vi "Convert Error Cluster to Table.vi"(11 "Error Codes":cluster{i32, string}[](array[cluster])) -> (2 "Code":i32[](array[numeric]), 3 "String":string[](array[string]))   [LabVIEW 2019, in "OPC UA Client System Explorer.lvlib"] (continued)
running the VI, this error occurs. The most likely cause is that you added a new session, and tried to use that new session in a running VI. Solution: Configure all session in LabVIEW project, then run the VI(s) that use those sessions."}, {-1074384541, "NI-XNET:  (Hex 0xBFF63163) You used an empty name for an XNET database object (database, cluster, ECU, frame, or signal). Empty name is not supported. Solution: Refer to NI-XNET help for IO names to review the required syntax for the name, and change your code to use that syntax."}, {-1074384540, "NI-XNET:  (Hex 0xBFF63164) You used a name for an XNET database object (such as frame or signal) that did not include a valid cluster selection. Solution: Refer to the NI-XNET help for the IO name that you are using, and use the syntax specified for that class, which includes the cluster selection."}, {-1074384539, "NI-XNET:  (Hex 0xBFF63165) Unsupported database file version. Solution: Use only database versions that are supported by this version of NI-XNET. Please see the NI-XNET documentation for information on which database versions are currently supported."}, {-1074384538, "NI-XNET:  (Hex 0xBFF63166) You used an empty name for the XNET Session. Empty name is not supported. Solution: Use a valid XNET session name from your LabVIEW project."}, {-1074384537, "NI-XNET:  (Hex 0xBFF63167) There is not enough message RAM on the FlexRay hardware to configure the data partition for the object(s). Solution: Please refer to the manual for limitations on the number of objects that can be created at any given time based on the payload length."}, {-1074384536, "NI-XNET:  (Hex 0xBFF63168) The FlexRay keyslot ID has been configured and a startup session has been created. Either the keyslot ID needs to be configured OR the startup session needs to be created. Both cannot exist at the same time. Solution: Choose a single method to configure startup sessions in your application."}, {-1074384535, "NI-XNET:  (Hex 0xBFF63169) An unsupported session was created. For example, stream output is not supported on FlexRay hardware. Solution: Only use supported sessions in your application."}, {-1074384528, "NI-XNET:  (Hex 0xBFF63170) An XNET session was created after starting the Interface. Only the Stream Input session in the subordinate mode can be created after the Interface has started. Solution: Create sessions prior to starting the XNET Interface in your application."}, {-1074384527, "NI-XNET:  (Hex 0xBFF63171) The Single Slot property was enabled on the XNET FlexRay Interface after the interface had started. Solution: Enable the Single Slot property prior to starting the XNET FlexRay Interface."}, {-1074384526, "NI-XNET:  (Hex 0xBFF63172) The FlexRay macrotick offset specified for XNET Create Timing Source is unsupported. Example: Specifying a macrotick offset greater than MacroPerCycle will result in this error. Solution: Specify a macrotick offset within the supported range for the cluster."}, {-1074384525, "NI-XNET:  (Hex 0xBFF63173) You used invalid syntax in the name of a database object (signal, frame, or ECU). For example, you may have specified a frame's name as <cluster>.<frame>, which is allowed in NI-XNET for C/C++, but not NI-XNET for LabVIEW. Solution: Use the string syntax specified in the help topic for the XNET I/O name class you are using."}, {-1074384524, "NI-XNET:  (Hex 0xBFF63174) A LIN schedule entry name is ambiguous, e.g., a schedule entry with the same name exists in another schedule. Solution: Specify the schedule name for the schedule entry using the required syntax."}, {-1074384523, "NI-XNET:  (Hex 0xBFF63175) A LIN schedule entry with the same name already exists in the schedule. Solution: Use another name for this schedule entry."}, {-1074384522, "NI-XNET:  (Hex 0xBFF63176) At least one of the frames in the session has an undefined identifier. Solution: Set the frame's \"Identifier (Slot)\" property before creating the session."}, {-1074384521, "NI-XNET:  (Hex 0xBFF63177) At least one of the frames in the session has an undefined payload length. Solution: Set the frame's \"Payload Length (in bytes)\" property before creating the session."}, {-1074384520, "NI-XNET:  (Hex 0xBFF63178) At least one of the signals in the session has an undefined start bit. Solution: Set the \"Start Bit\" property of the signal before creating the session."}, {-1074384519, "NI-XNET:  (Hex 0xBFF63179) At least one of the signals in the session has an undefined number of bits. Solution: Set the \"Number of Bits\" property of the signal before creating the session."}, {-1074384518, "NI-XNET:  (Hex 0xBFF6317A) At least one of the signals in the session has an undefined byte order. Solution: Set the \"Byte Order\" property of the signal before creating the session."}, {-1074384517, "NI-XNET:  (Hex 0xBFF6317B) At least one of the signals in the session has an undefined data type. Solution: Set the \"Data Type\" property of the signal before creating the session."}, {-1074384516, "NI-XNET:  (Hex 0xBFF6317C) At least one of the subframes in the session has an undefined multiplexer value. Solution: Set the \"Multiplexer Value\" property of the subframe before creating the session."}, {-1074384515, "NI-XNET:  (Hex 0xBFF6317D) You provided an invalid index to Write (State LIN Schedule Change). Solution: Use a number from 0 to N-1, where N is the number of LIN schedules returned from the cluster property LIN Schedules. If you are using LabVIEW, the string for the number must be decimal (not hexadecimal)."}, {-1074384514, "NI-XNET:  (Hex 0xBFF6317E) You provided an invalid name to Write (State LIN Schedule Change). Solution: Use a valid LIN schedule name returned from the cluster property LIN Schedules, or the session property Interface LIN Schedules. You can use the short name (schedule only) or long name (schedule plus database and cluster)."}, {-1074384513, "NI-XNET:  (Hex 0xBFF6317F) You provided an invalid active index for the session property.\nFor LabVIEW, this is the Frame:Active in the session property node.\nFor C/C++, this is the ActiveIndex parameter of nxGetSubProperty/nxSetSubProperty.\nSolution: Use a number from 0 to N-1, where N is the number of items in the session's List property. If you are using LabVIEW, the string for the number must be decimal (not hexadecimal)."}, {-1074384512, "NI-XNET:  (Hex 0xBFF63180) You provided an invalid name for Frame:Active of the session property node. Solution: Use a valid item name from the session's List property. You can use the short name (frame or signal only) or long name (frame/signal plus database and cluster)."}, {-1074384511, "NI-XNET:  (Hex 0xBFF63181) The database you are using requires using PDUs, and the operation is ambiguous with respect to PDUs. Example: You are trying to get the frame parent of the signal, but the PDU in which the signal is contained is referenced in multiple frames."}, {-1074384510, "NI-XNET:  (Hex 0xBFF63182) A PDU with the same name already exists in the cluster. Solution: Use another name for this PDU."}, {-1074384509, "NI-XNET:  (Hex 0xBFF63183) You are trying to assign start bits or update bits to PDUs referenced in a frame, but the number of elements in this array is different than the number of referenced PDUs. Solution: Use the same number of elements in the array as in the PDU references array."}, {-1074384508, "NI-XNET:  (Hex 0xBFF63184) The configuration of this object requires using advanced PDUs, which the given protocol does not support. Solution: You cannot use this object in the given protocol."}, {-1074384507, "NI-XNET:  (Hex 0xBFF63185) The maximum number of PDUs has been exceeded. Solution: Use fewer PDUs in your sessions."}, {-1074384506, "NI-XNET:  (Hex 0xBFF63186) This mode value is not currently supported. Solution: Use a valid value."}, {-1074384505, "NI-XNET:  (Hex 0xBFF63187) The firmware image on your XNET hardware is corrupted. Solution: Update the firmware of this XNET hardware in MAX."}, {-1074384504, "NI-XNET:  (Hex 0xBFF63188) The firmware version of your XNET hardware is not in sync with your host computer. Solution: Update the firmware of this XNET hardware in MAX."}, {-1074384503, "NI-XNET:  (Hex 0xBFF63189) The firmware version of your XNET C Series module is not in sync with the NI-XNET software on your remote target. Solution: Update the NI-XNET software on the remote target."}, {-1074384502, "NI-XNET:  (Hex 0xBFF6318A) The terminal you are trying to use is already in use. Only one connection per terminal is allowed.  Solution: Disconnect the terminal that is already in use."}, {-1074384501, "NI-XNET:  (Hex 0xBFF6318B) You need to install a supported version of NI-DAQmx for your XNET C Series module to work correctly with your Compact DAQ system. Solution: Check the NI-XNET readme file for supported versions of the NI-DAQmx driver software."}, {-1074384500, "NI-XNET:  (Hex 0xBFF6318C) Unable to create the requested route. This may be caused by a routing conflict or an invalid terminal name. Solution: Fix invalid terminal names, such as a blank string. Since NI-XNET relies on the NI-DAQmx driver software to create routes on Compact DAQ chassis, use DAQmx to resolve routing conflicts."}, {-1074384499, "NI-XNET:  (Hex 0xBFF6318D) You attempted to transmit a go to sleep frame (by setting the LIN Sleep mode to Remote Sleep) on a LIN interface configured as slave.  In conformance with the LIN protocol standard, only an interface configured as master may transmit a go to sleep frame."}, {-1074384498, "NI-XNET:  (Hex 0xBFF6318E) You attempted to set properties related to Sleep and Wakeup when the FlexRay cluster defined in the Fibex file does not support it. Solution: Edit the Fibex file used in your application to include all relevant cluster wakeup attributes."}, {-1074384497, "NI-XNET:  (Hex 0xBFF6318F) A LIN diagnostic schedule change requires the diagnostic schedule to be defined in the database. Solution: Define the diagnostic schedule in the database."}, {-1074384494, "NI-XNET:  (Hex 0xBFF63192) The data payload written for a diagnostic frame for transmit does not conform to the LIN transport layer specification.  Solution: Ensure the data payload for a diagnostic frame conforms to the transport layer specification."}, {-1074384493, "NI-XNET:  (Hex 0xBFF63193) An error occurred within the NI-XNET example code for logfile access (TDMS). Solution: For LabVIEW, the subVI with the error is shown as the source, and you can open that subVI to determine the cause of the problem. For other programming languages, review the source code for the logfile example to determine the cause of the problem."}, {-1074384384, "NI-XNET:  (Hex 0xBFF63200) You attempted to write a LIN schedule and use a stream output replay timing mode concurrently. You can only use the stream output immediate timing mode cuncurrently with the LIN scheduler."}, {-1074384383, "NI-XNET:  (Hex 0xBFF63201) You attempted to create a session that is incompatible with the LIN interface personality (master or slave), or set the LIN interface personality to one that is incompatible with a session already created for it. For example, setting the LIN interface to slave after creating a stream output session will report this error, because only LIN interface as master supports stream output."}, {-1074384382, "NI-XNET:  (Hex 0xBFF63202) You attempted to save an LDF or DBC database, but the passed reference is not a database cluster. Solution: A cluster reference must be used to specify the cluster you want to export."}, {-1074384381, "NI-XNET:  (Hex 0xBFF63203) You tried to assign the same interface name twice. This is not permitted. Solution: Assign a unique name to an interface."}, {-1074384380, "NI-XNET:  (Hex 0xBFF63204) Transceiver cable hardware revision is too new. The current driver does not support this transceiver cable. Solution: Upgrade the NI-XNET driver."}, {-1074384379, "NI-XNET:  (Hex 0xBFF63205) Transceiver cable image revision is too new. The current driver does not support this transceiver cable. Solution: Upgrade the NI-XNET driver or downgrade the image on the transceiver cable."}, {-1074384378, "NI-XNET:  (Hex 0xBFF63206) The property does not apply to this type of hardware. For example, a dongle revision property cannot be accessed on an XNET device that does not support Transceiver Cables. Solution: Do not apply the property to this type of hardware."}, {-1074384377, "NI-XNET:  (Hex 0xBFF63207) Exporting cluster into the specified database type failed. Solution: Ensure the database configuration is complete. Refer to the standard documentation for the related file format."}, {-1074384376, "NI-XNET:  (Hex 0xBFF63208) A J1939 input queue overflowed. Reading large J1939 frames can make  the queue overflow, and the Read function delivers fewer frames then specified.  Solution: Call the Read function again to read the remaining frames."}, {-1074384375, "NI-XNET:  (Hex 0xBFF63209) You are trying to transmit a non-J1939 frame with more than 8 bytes. Only J1939 frames can use the J1939 transport protocol.  Solution: Verify the transport protocol property on the frame in  the database."}, {-1074384374, "NI-XNET:  (Hex 0xBFF6320A) You are trying to transmit a J1939 frame, but no J1939 address is assigned to the session. Solution: Set the address using the J1939 address property."}, {-1074384373, "NI-XNET:  (Hex 0xBFF6320B) The received J1939 TP.CM_CTS message has the wrong total size."}, {-1074384372, "NI-XNET:  (Hex 0xBFF6320C) The next packet value of the received J1939 TP.CM_CTS message is larger than the total number of packets."}, {-1074384371, "NI-XNET:  (Hex 0xBFF6320D) The received J1939 TP.CM_CTS message has a number of packets of 0, but the next packet number is not 255."}, {-1074384370, "NI-XNET:  (Hex 0xBFF6320E) The received J1939 TP.CM_CTS message has a next packet value of 0."}, {-1074384369, "NI-XNET:  (Hex 0xBFF6320F) The received J1939 TP.CM_CTS message does not have the same PGN as in the TP.CM_RTS message."}, {-1074384368, "NI-XNET:  (Hex 0xBFF63210) Received unexpected sequence number in the J1939 TP.DT message."}, {-1074384367, "NI-XNET:  (Hex 0xBFF63211) More Packets are requested than allowed in the J1939 TP.CM_CTS message."}, {-1074384366, "NI-XNET:  (Hex 0xBFF63212) J1939 Timeout T1 while waiting for data."}, {-1074384365, "NI-XNET:  (Hex 0xBFF63213) J1939 Timeout T2 while waiting for data."}, {-1074384364, "NI-XNET:  (Hex 0xBFF63214) J1939 Timeout T3 while waiting for TP.CM_CTS or TP.CM_EndOfMsgAck."}, {-1074384363, "NI-XNET:  (Hex 0xBFF63215) J1939 Timeout T4 while waiting for next CTS MSG."}, {-1074384362, "NI-XNET:  (Hex 0xBFF63216) Received wrong DLC in the J1939 TP.CM_RTS message. DLC must be 8."}, {-1074384361, "NI-XNET:  (Hex 0xBFF63217) Received wrong DLC in the J1939 TP.CM_CTS message. DLC must be 8."}, {-1074384360, "NI-XNET:  (Hex 0xBFF63218) Received wrong DLC in the J1939 TP.CM_BAM message. DLC must be 8."}, {-1074384359, "NI-XNET:  (Hex 0xBFF63219) Received wrong DLC in the J1939 TP.DT message. DLC must be 8."}, {-1074384358, "NI-XNET:  (Hex 0xBFF6321A) Received wrong DLC in the J1939 TP.CM_Abort message. DLC must be 8."}, {-1074384357, "NI-XNET:  (Hex 0xBFF6321B) Received wrong DLC in the J1939 TP.CM_EndOfMsgAck message. DLC must be 8."}, {-1074384356, "NI-XNET:  (Hex 0xBFF6321C) Received wrong PGN in the J1939 TP.CM_Abort message."}, {-1074384355, "NI-XNET:  (Hex 0xBFF6321D) Internal error occurred for send TP.CM_CTS Hold Message."}, {-1074384354, "NI-XNET:  (Hex 0xBFF6321E) Invalid total message size in J1939 TP.CM_RTS message. Expect 9..1785."}, {-1074384353, "NI-XNET:  (Hex 0xBFF6321F) Total number of packets in received J1939 TP.CM_RTS message must be greater than 1."}, {-1074384352, "NI-XNET:  (Hex 0xBFF63220) Reserved data bytes in J1939 received message are not BFF63FF."}, {-1074384351, "NI-XNET:  (Hex 0xBFF63221) Not enough system resources for the J1939 Transport Protocol."}, {-1074384350, "NI-XNET:  (Hex 0xBFF63222) Received J1939 TP.CM_Abort message with reason ActiveConnection: Already in one or more connection managed sessions and cannot support another."}, {-1074384349, "NI-XNET:  (Hex 0xBFF63223) Received J1939 TP.CM_Abort message with reason NotEnoughSystemResources: System resources were needed for another task, so this connection managed session was terminated."}, {-1074384348, "NI-XNET:  (Hex 0xBFF63224) Received J1939 TP.CM_Abort message with reason Timeout: A timeout occurred, and this is the connection abort to close the session."}, {-1074384347, "NI-XNET:  (Hex 0xBFF63225) Received J1939 TP.CM_Abort message with reason CtsReceived: CTS messages received when data transfer is in progress."}, {-1074384346, "NI-XNET:  (Hex 0xBFF63226) Received J1939 TP.CM_Abort message with reason MaxRetransmit: Maximum retransmit request limit reached."}, {-1074384345, "NI-XNET:  (Hex 0xBFF63227) Remote communication with the LabVIEW RT target failed because the host and target versions of NI-XNET are different. Solution: On the target, install the same NI-XNET version that is installed on the host."}, {-1074384344, "NI-XNET:  (Hex 0xBFF63228) The CAN frame I/O mode is higher than the CAN cluster  I/O mode. This frame cannot be transmitted on the network. Solution: Change the frame or cluster I/O mode."}, {-1074384343, "NI-XNET:  (Hex 0xBFF63229) The current driver cannot update the firmware on your hardware. Solution: Ask National Instruments for compatible driver software."}, {-1074384342, "NI-XNET:  (Hex 0xBFF6322A) You are trying to use the CAN Transmit I/O Mode (TxIoMode) property in an unsupported interface mode. Solution: You can use this property in only non-ISO or ISO Legacy mode."}, {-1074384341, "NI-XNET:  (Hex 0xBFF6322B) You are trying to use the XS Transceiver Cable on unsupported hardware. This currently requires a PXIe-8510 board."}, {-1074384340, "NI-XNET:  (Hex 0xBFF6322C) You are trying to use a database alias name that contains an invalid character (for example, a comma)."}, {-1074384339, "NI-XNET:  (Hex 0xBFF6322D) You are trying to use a database filepath that contains an invalid character (for example, a comma)."}, {-1074384338, "NI-XNET:  (Hex 0xBFF6322E) You are trying to use CAN FD with a non-HS/FD port. CAN FD is supported with High Speed CAN only."}, {-1074384337, "NI-XNET:  (Hex 0xBFF6322F) An unconditional LIN schedule entry is incorrectly configured. To fix this issue, reference only one frame in this entry."}, {-1074384336, "NI-XNET:  (Hex 0xBFF63230) An event LIN schedule entry has no collision resolving schedule assigned. To fix this issue, assign a schedule to the schedule entry."}, {-1074384335, "NI-XNET:  (Hex 0xBFF63231) You have connected your USB device to a port that supports only Full Speed (USB 1.1). NI-XNET USB devices require at least High Speed (USB 2.0+) support for correct operation."}, {-1074384334, "NI-XNET:  (Hex 0xBFF63232) You added two or more frames with different payload sizes to the same LIN event-triggered schedule entry. Use an equal payload length for all event-triggered frames in an event-triggered schedule entry."}, {-1074384333, "NI-XNET:  (Hex 0xBFF63233) You added two or more frames with different checksum types to the same event-triggered schedule entry. The LIN checksum type is determined by the LIN protocol version of the ECU transmitting the frame. Solution: Use the same checksum model for all event-triggered frames in an event-triggered schedule entry."}, {-1074384332, "NI-XNET:  (Hex 0xBFF63234) The versions of the NI-XNET device driver and Compact RIO driver are incompatible. Solution: Install drivers listed in the Recommended Software Set."}, {-1074384331, "NI-XNET:  (Hex 0xBFF63235) The module support for this slot is missing features required for the NI-XNET driver to be able to communicate with the module. Solution: Load a bitfile to the chassis that contains support for NI-XNET modules for the occupied slots."}, {-1074384330, "NI-XNET:  (Hex 0xBFF63236) The interface you have attempted to use with NI-XNET Compatibility Library is already in use by NI-XNET.  Solution: Stop all applications running on the interface, or select one not in use by NI-XNET sessions."}, {-1074384329, "NI-XNET:  (Hex 0xBFF63237) The interface you have attempted to use with NI-XNET is already in use by NI-XNET Compatibility Library.  Solution: Stop all applications running on the interface, or select one not in use by the NI-XNET Compatibility Library."}, {-1074384328, "NI-XNET:  (Hex 0xBFF63238) Byte array signals are not allowed for this session type or function. Solution: Select only numeric signals for the session."}, {-1074384327, "NI-XNET:  (Hex 0xBFF63239) Mixing of byte array signals and numeric signals is not allowed for this session type. Solution: Select only numeric signals or byte array signals for the session."}, {-1074384326, "NI-XNET:  (Hex 0xBFF6323A) Only one byte array signal is allowed for this session type or function. Solution: Select only one byte array signal for the session."}, {-1074384325, "NI-XNET:  (Hex 0xBFF6323B) The feature you have attempted to use is not supported. Solution: Use an alternate feature that is supported."}, {-1074384324, "NI-XNET:  (Hex 0xBFF6323C) The specified property is write-only and is therefore not readable. Solution: Do not read write-only properties."}, {-1074384323, "NI-XNET:  (Hex 0xBFF6323D) FPGA download is not possible because the board is in use by an application. Solution: Stop all NI-XNET applications before executing FPGA download."}, {-1074384322, "NI-XNET:  (Hex 0xBFF6323E) The trigger timestamp cannot be read, because the trigger source is not connected. Solution: Connect the TimeTrigger to a valid source before reading the timestamp."}, {-1074384321, "NI-XNET:  (Hex 0xBFF6323F) The trigger timestamp cannot be read, because another operation is reading the timestamp. Solution: Perform only one trigger timestamp read at a time."}, {-1074384320, "NI-XNET:  (Hex 0xBFF63240) The wait did not complete, because it was aborted. This typically occurs when the XNET session is closed while a wait is in progress. Solution: Allow the wait to finish before closing the XNET session."}, {-1074384319, "NI-XNET:  (Hex 0xBFF63241) The future time trigger cannot be generated, because the trigger destination is not connected. Solution: Connect the TimeTrigger to a valid destination before generating the future time trigger."}, {-1074384318, "NI-XNET:  (Hex 0xBFF63242) The log file could not be created because it already exists. Solution: Specify a different file name or choose a mode that allows overwriting the file."}, {-1074384317, "NI-XNET:  (Hex 0xBFF63243) Could not create or replace the log file. This can happen if there are insufficient file permissions at the specified location or invalid file path syntax."}, {-1074384316, "NI-XNET:  (Hex 0xBFF63244) You cannot read data using XNET Read after a session has been started with logging enabled."}, {-1074384315, "NI-XNET:  (Hex 0xBFF63245) A problem has been detected with the firmware on the device. Solution: Stop your application and try disabling/re-enabling the driver in Device Manager. If the problem persists, contact National Instruments."}, {-1074384314, "NI-XNET:  (Hex 0xBFF63246) A write queue overflowed for a session that has not been started. Solution: Write less data before starting the session, or write data after the session has already been started."}, {-1074384313, "NI-XNET:  (Hex 0xBFF63247) The total size of the data to be transmitted is larger than the internal write queue. Solution: Write less data at a time."}, {-1074384312, "NI-XNET:  (Hex 0xBFF63248) The requested number of packets do not fit in the current queue. Solution: Increase the queue size or decrease the number of packets to read."}, {-1074384311, "NI-XNET:  (Hex 0xBFF63249) You wrote a frame whose payload length is smaller than the minimum payload size allowed. Solution: Never write fewer payload bytes than the minimum allowed size for the session."}, {-1074384310, "NI-XNET:  (Hex 0xBFF6324A) The XNET endpoint on this port cannot start while the Port Mode is set to Tap. The endpoint has no access to data while in this mode. Solution: Set the Port Mode to Direct to have full use of the XNET endpoint."}, {-1074384309, "NI-XNET:  (Hex 0xBFF6324B) The future time trigger cannot be generated because a previously scheduled future time trigger is still pending. Solution: Wait until the previously scheduled future time trigger occurs, or cancel the pre-existing trigger by disconnecting the time trigger resource."}, {-1074384308, "NI-XNET:  (Hex 0xBFF6324C) The desired time to generate the future time trigger has already elapsed. Solution: Schedule the future time trigger for a point in time further into the future."}, {-1074384307, "NI-XNET:  (Hex 0xBFF6324D) The network time cannot be adjusted while this clock is a slave (i.e., not grandmaster). Solution: Wait until the port state is no longer set to slave or configure this clock as a grandmaster."}, {-1074384306, "NI-XNET:  (Hex 0xBFF6324E) Output sessions must be created using an interface's endpoint path. Solution: Change the interface to use the endpoint path (e.g., use the interface name that does not contain \"/monitor\")."}, {-1074384305, "NI-XNET:  (Hex 0xBFF6324F) The time protocol cannot be used while the Port Mode is set to Tap. Solution: If Tap mode is desired, disable the time protocol on both ports of the Tap pair before switching to Tap mode. If usage of the time protocol is desired, set the Port Mode to Direct before enabling the time protocol."}, {-1074384304, "NI-XNET:  (Hex 0xBFF63250) You cannot write data while the XNET session is started and the link is down. Solution: Ensure the link is up prior to writing data. You can use the Operational Status property to query the current link state."}, {-1074384303, "NI-XNET:  (Hex 0xBFF63251) Device reset is not possible since the board is in use by an application. Solution: Stop all NI-XNET applications before executing a device reset."}, {-1074384302, "NI-XNET:  (Hex 0xBFF63252) You cannot start an NI-XNET application while a device reset is in progress. Solution: Complete the device reset before starting any NI-XNET applications."}, {-1074384301, "NI-XNET:  (Hex 0xBFF63253) You wrote a frame whose frame type value is not valid. Solution: Encode the frame with frame type value that is supported by NI-XNET."}, {-1074384300, "NI-XNET:  (Hex 0xBFF63254) The data path you have attempted to use is already in use by another session. Solution: Stop the other application using the desired data path, or select a data path not in use by NI-XNET sessions."}, {-1074384299, "NI-XNET:  (Hex 0xBFF63255) The timescale value is invalid. Solution: Use a valid value."}, {-1074384298, "NI-XNET:  (Hex 0xBFF63256) A hardware error has occurred while reading the Port MAC address. Solution: Reset this XNET hardware in MAX."}, {-1074384297, "NI-XNET:  (Hex 0xBFF63257) You cannot write to the Time Sync Protocol property while the Port Mode is set to Tap. Solution: Do not write to this property while ports are configured to use Tap mode. To configure the Time Sync Protocol property, set the Port Mode to Direct before writing to this property."}, {-1074384296, "NI-XNET:  (Hex 0xBFF63258) The buffer is not large enough to contain the requested path."}, {-1074384295, "NI-XNET:  (Hex 0xBFF63259) A NULL pointer or an empty string was passed when requesting a path."}, {1073098816, "NI-XNET:  (Hex 0x3FF63040) The CAN FD baud rate you supplied exceeds the capabilities the transceiver manufacturer specified. In our internal testing, we have found this baud rate to run, but bus errors may be detected or generated during communication. Refer to the NI-XNET CAN Hardware Overview section in the NI-XNET Hardware and Software Manual for more information."}, {1073098885, "NI-XNET:  (Hex 0x3FF63085) There is a warning from importing the database file. For details, refer to the log files found in %LOCALAPPDATA%\\National Instruments\\NI-XNET\\log. Please note that this location may be hidden on your computer."}, {1073098886, "NI-XNET:  (Hex 0x3FF63086) The database file has been imported, but it was not created by the XNET Editor or using the XNET API. Saving the database file with the XNET API or XNET Editor may lose information from the original file."}, {1073098887, "NI-XNET:  (Hex 0x3FF63087) The database file was not created by the XNET Editor or using the XNET API. Additionally, there is another warning. For details, refer to the import log file nixnetfx-log.txt under %LOCALAPPDATA%\\National Instruments\\NI-XNET\\log. Please note that this location may be hidden on your computer."}, {1073099057, "NI-XNET:  (Hex 0x3FF63131) Close Database returns a warning instead of an error when an invalid reference is passed to the function."}, {1073099058, "NI-XNET:  (Hex 0x3FF63132) You are retrieving signals from a frame that uses advanced PDU configuration. The signal start bit is given relative to the PDU, and it may be different than the start bit relative to the frame."}, {-307998, "NI VeriStand: The SLSC chassis name or IP address/hostname is empty."}, {-307997, "NI VeriStand: VeriStand does not support SLSC on targets running VxWorks."}, {-307996, "NI VeriStand: SLSC module not found in the specified slot. Please check your SLSC hardware and make sure the custom device is inserted in the correct slot."}, {-307995, "NI VeriStand: VeriStand engine failed to retrieve data from the SLSC chassis status loop within the specified timeout."}, {-307994, "NI VeriStand: The specified parameter cannot be found."}, {-307993, "NI VeriStand: The parameter dimension does not match the parameter default value length."}, {-307992, "NI VeriStand: The specified operation cannot be completed. There is no project file currently open."}, {-307991, "NI VeriStand: A real-time sequence parameter assignment has an invalid data type. The data type of the value assigned to the parameter must match the parameter data type."}, {-307990, "NI VeriStand: A system definition channel has been mapped to two or more real-time sequence parameters that are not the same data type. A channel can only be mapped to multiple parameters if they share the same data type."}, {-307989, "NI VeriStand: The specified parameter assignment is not valid. The channel mapped to the parameter could not be found in the system."}, {-307988, "NI VeriStand: The specified real-time sequence contains one or more errors which caused it to fail to compile."}, {-307987, "NI VeriStand: One or more real-time sequence parameters with a by-reference evaluation was not mapped to. You must assign a value to all real-time sequence parameters that have a by-reference evaluation type."}, {-307986, "NI VeriStand: The specified parameter assignment is not valid. The real-time sequence parameter does not exist."}, {-307985, "NI VeriStand: The sequence did not complete the timestep within the specified timeout in milliseconds. This could be due to a sequence that contains too much processing or an infinite loop that does not yield. To resolve this issue, evaluate the timing of your sequence or increase the timeout."}, {-307984, "NI VeriStand: The stimulus profile session already is deployed."}, {-307983, "NI VeriStand: The sequence containing the specified variable is currently running. You cannot probe a variable value while a sequence is running."}, {-307982, "NI VeriStand: The stimulus profile session is not deployed."}, {-307981, "NI VeriStand: The stimulus profile session does not contain a sequence with the specified name."}, {-307980, "NI VeriStand: The specified stimulus profile session is locked. A stimulus profile session must be unlocked before any sequences in the session can be controlled."}, {-307974, "NI VeriStand: Error provider received an unexpected configuration. Verify the error provider is implemented correctly and the errors can be handled by the error provider."}, {-307973, "NI VeriStand: Error provider received an electrical error with an unexpected number of signals. Verify the error provider is implemented correctly and all errors contain the correct number of signals."}, {-307972, "NI VeriStand: Error provider received an electrical error that contains a signal it cannot handle. Verify the error provider is implemented correctly and all errors contain the correct signals."}, {-307971, "NI VeriStand: A channel cannot have child items."}, {-307970, "NI VeriStand: An inline custom device attempted to access invalid data in the VeriStand Engine. The inline custom device attempted to read or write data using an invalid reference, or a reference that did not have the read or write access required for that operation."}, {-307952, "NI VeriStand: Two or more models (.mdl files) are using the same VeriStand Server port at the same time. The VeriStand Server can only run one model instance at a time."}, {-307951, "NI VeriStand: NI VeriStand requires that a model (.mdl file) be compiled before it can run on a real-time (RT) target."}, {-307950, "NI VeriStand: Unable to connect to the NI VeriStand Model Simulation Server."}, {-307949, "NI VeriStand: The selected model (.mdl file) is invalid.  Verify that the model can be compiled and run properly, that you have added an NIVeriStandSignalProbe block to it, and that the stop time is set to inf."}, {-307948, "NI VeriStand: Connection refused. Unable to establish a connection between the VeriStand  Model Simulation Server and client. The NI VeriStand MDL client version is incompatible with the currently loaded NI VeriStand  Model Simulation  Server."}, {-307933, "NI VeriStand: Attempted to write to a read-only property."}, {-307932, "NI VeriStand: The formula type must depend on variables."}, {-307931, "NI VeriStand: Model execution order group cannot be empty."}, {-307930, "NI VeriStand: A node name cannot be an empty string."}, {-307929, "NI VeriStand: The mapping definition is invalid. The source channel must be readable, the destination channel must be writable, and both channels cannot be part of the stimulus generator."}, {-307928, "NI VeriStand: Found an existing FPGA target with the same RIO address configuration."}, {-307927, "NI VeriStand: Invalid argument. The node reference is not a valid channel."}, {-307926, "NI VeriStand: This node already exists in the system."}, {-307925, "NI VeriStand: The specified node is not compatible with this operation."}, {-307917, "NI VeriStand: A stimulus profile generator contains channel mappings for channels on a different target than the target on which the generator will execute. A generator can only map to channels on the target on which it will execute. Confirm that the generator is not mapped to channels from different targets, or that the generator does not specify an execution target that is different than one of the channel mappings."}, {-307916, "NI VeriStand: A stimulus profile generator contains a Set Variable step that attempts to set a variable on another target. A Set Variable step only can set a variable on the same target as the generator containing the step."}, {-307915, "NI VeriStand: The operation could not be completed. A stimulus profile currently is running."}, {-307914, "NI VeriStand: The specified CSV file does not contain a <b>Timestamp</b> column. The file you specify must have a <b>Timestamp</b> column that contains values in milliseconds."}, {-307913, "NI VeriStand: The number of stimulus generators exceeds the maximum specified on the <b>Stimulus Configuration</b> page of the <b>System Explorer</b> window. To correct this error, reduce the number of total stimulus generators used in the stimulus profile. You also can increase the number of generators using the <b>Stimulus Configuration</b> page of the <b>System Explorer</b> window."}, {-307912, "NI VeriStand: The number of data points exceeds the maximum analysis buffer size specified on the <b>Stimulus Configuration</b> page of the <b>System Explorer</b> window. To correct this error, reduce the number of data points in the stimulus profile. You also can increase the maximum analysis buffer size specified in the <b>Stimulus Configuration</b> page of the <b>System Explorer</b> window."}, {-307911, "NI VeriStand: Unable to start stimulus profile generation. One or more calibration files are not found."}, {-307910, "NI VeriStand: Unable to start stimulus profile generation. CAN logging requires that the CAN Bus Monitor is running."}, {-307909, "NI VeriStand: Unable to start stimulus profile generation. Stimulus profile file contains invalid profile steps or incorrect timing."}, {-307908, "NI VeriStand: The stimulus profile manager currently is reserved by a client."}, {-307907, "NI VeriStand: Multi-point data does not have the correct timing. The data must start at time 0 and increment at a multiple of Delta t value."}, {-307906, "NI VeriStand: Timeout occurred while writing data to the analysis buffer."}, {-307905, "NI VeriStand: Timeout occurred while writing data to the auxiliary buffer."}, {-307904, "NI VeriStand: A stimulus profile failed to compile correctly. The profile might reference invalid channels. Verify that the stimulus profile links to valid channels."}, {-307903, "NI VeriStand: The number of data points exceeds the maximum auxiliary buffer size specified on the <b>Stimulus Configuration</b> page of the <b>System Explorer</b> window. To correct this error, reduce the number of data points in the stimulus profile. You also can increase the maximum auxiliary buffer size specified in the <b>Stimulus Configuration</b> page of the <b>System Explorer</b> window."}, {-307902, "NI VeriStand: The specified stimulus profile is empty. It contains no compiled steps."}, {-307901, "NI VeriStand: The number of compiled stimulus generator steps exceeds the maximum specified on the <b>Stimulus Configuration</b> page of the <b>System Explorer</b> window. To correct this error, reduce the number of steps in the stimulus generator. You also can increase the maximum number of steps per generator using the <b>Stimulus Configuration</b> page."}, {-307900, "NI VeriStand: The number of generator mappings exceeds the maximum specified on the <b>Stimulus Configuration</b> page of the <b>System Explorer</b> window. To correct this error, reduce the number of mapped channels. You also can increase the maximum number of mappings per generator using the <b>Stimulus Configuration</b> page."}, {-307891, "NI VeriStand: VeriStand only supports devices whose calibration password is the default value. Use NI MAX or the NI System Configuration API to reset the calibration password on the device to the default value."}, {-307890, "NI VeriStand: The CJC source specified for a thermocouple scale is invalid."}, {-307889, "NI VeriStand: A lookup table scale mapped to a channel(s) is empty. Remove the mapping or update the scale to contain pairs of pre-scaled values and the corresponding values to which to scale them, and then try to deploy the system definition again."}, {-307888, "NI VeriStand: A polynomial scale mapped to a channel(s) does not have reverse coefficients defined. Remove the mapping or update the scale to contain reverse coefficients, and then try to deploy the system definition again."}, {-307887, "NI VeriStand: A polynomial scale mapped to a channel(s) does not have coefficients defined. Remove the mapping or update the scale to contain coefficients, and then try to deploy the system definition again."}, {-307886, "NI VeriStand: The CJC channel source for a thermocouple scale is not on the same target as the channel to which this scale is applied."}, {-307885, "NI VeriStand: The scale type you specified is invalid. Scale type can have only the following values 0: Polynomial. 1: Thermocouple. 2: Lookup table."}, {-307884, "NI VeriStand: A polynomial scale cannot contain more than ten coefficients. Reduce the number of coefficients to ten or fewer."}, {-307883, "NI VeriStand: Cannot deploy project because the system definition file contains scales but the project does not contain a channel calibration file (.nivscf). Either delete the scales from the system definition file and redeploy or add a .nivscf file to the project under the <B>Calibrations</B> node in the <B>Project Explorer</B> window."}, {-307882, "NI VeriStand: Cannot use Channel Calibration tool/API because this project does not contain a channel calibration file (.nivscf). If you want to use the Channel Calibration tool/API, add a .nivscf file to the project under the <B>Calibrations</B> node in the <B>Project Explorer</B> window. Otherwise, you can use the legacy Channel Scaling and Calibration Tool/API instead of the Channel Calibration tool/API."}, {-307881, "NI VeriStand: Cannot use legacy Channel Scaling and Calibration tool/API because this project contains calibration features from the new Channel Calibration tool/API introduced in NI VeriStand 2012. This error occurs because the project contains a channel calibration file (.nivscf). If you want to use the legacy Channel Scaling and Calibration tool, delete the .nivscf file under the <B>Calibrations</B> node in the <B>Project Explorer</B> window and redeploy. Otherwise, use the Channel Calibration Tool/API instead of the legacy Channel Scaling and Calibration tool/API."}, {-307872, "NI VeriStand: There was an error downloading one or more of the requested files. Please use the errors parameter for more detaield information."}, {-307871, "NI VeriStand: Cannot retrieve information for the specified log file. Ensure the session name and filename are correct."}, {-307870, "NI VeriStand: A compatible version of NI DIAdem is not installed. You must have NI DIAdem installed to load data in NI DIAdem."}, {-307869, "NI VeriStand: Data was lost while logging data. Samples may be missing from the log file. Start and stop triggers could also have missed data to evaluate."}, {-307868, "NI VeriStand: The specified trigger condition contains syntax errors."}, {-307867, "NI VeriStand: The specified data logging session name is already in use. Specify a unique data logging session name."}, {-307866, "NI VeriStand: An error occurred while logging data. Refer to the error description for more information."}, {-307865, "NI VeriStand: The specified data logging session does not exist."}, {-307864, "NI VeriStand: The specified log file path is not valid. It might include invalid tags."}, {-307863, "NI VeriStand: The specified property value is not a valid data type for a TDMS property."}, {-307862, "NI VeriStand: The specified data logging configuration resulted in a buffer size that exceeds the maximum allowed size. Reduce the buffer size by reducing the pre-trigger time, the logging rate, or the number of logged channels in the data logging configuration."}, {-307861, "NI VeriStand: The data logging configuration is invalid. One or more specified channels does not exist."}, {-307860, "NI VeriStand: The specified trigger channel does not exist."}, {-307853, "NI VeriStand: The VeriStand Gateway was unable to establish a connection with the target. Confirm that the target is running and that the VeriStand Engine successfully has started. If you still cannot connect to the target, use MAX to reinstall the NI VeriStand Run-Time Engine to the target."}, {-307852, "NI VeriStand: The specified dependent file is contained within an LLB, but the destination path on the target is not contained in an LLB. Individual files cannot be copied out of an LLB. The destination path on the target must have an LLB as the parent of the dependent file."}, {-307851, "NI VeriStand: One or more system definition file dependency files differ from the originally imported version. This might cause unexpected behavior or errors. Cancel the current operation and resolve any conflicts in the <b>System Explorer</b> window."}, {-307850, "NI VeriStand: The target cannot be reached. Verify that the Ethernet cable is connected to the real-time (RT) target and that the RT target is enabled and running."}, {-307832, "NI VeriStand: The depending file path is improperly formed or cannot be found."}, {-307831, "NI VeriStand: Unable to save file to the specified path."}, {-307830, "NI VeriStand: The channel dimension does not match the channel default value length."}, {-307829, "NI VeriStand: The specified node cannot be found."}, {-307828, "NI VeriStand: This dependency does not refer to a valid item. The item may have been deleted. To correct the dependency, re-add the invalid item and click <B>Update Dependencies</B> in this dialog box, or select a different dependency."}, {-307827, "NI VeriStand: The specified item is not an expected type inside the system storage hierarchy."}, {-307826, "NI VeriStand: The specified item is not an alias for a channel."}, {-307825, "NI VeriStand: The specified item is not a channel."}, {-307824, "NI VeriStand: The specified item is not a waveform."}, {-307800, "NI VeriStand: A procedure failed to compile correctly and cannot be executed."}, {-307785, "NI VeriStand: No error provider exists to handle the error signals."}, {-307784, "NI VeriStand: STI file is not valid."}, {-307783, "NI VeriStand: The data structure contains a dependencies cycle."}, {-307782, "NI VeriStand: The channel cannot be found in the specified log file"}, {-307781, "NI VeriStand: The channel group cannot be found in the specified log file."}, {-307780, "NI VeriStand: The specified feature is supported only if the gateway is running on the localhost machine."}, {-307756, "NI VeriStand: Internal error: The DAQmx waveform producer received a command which was not declared as a publicly available."}, {-307755, "NI VeriStand: The specified operation is not permitted while recording a macro."}, {-307754, "NI VeriStand: Serialization error. Unable to save macro."}, {-307753, "NI VeriStand: The specified operation is not permitted unless playing a macro."}, {-307752, "NI VeriStand: The specified operation is not permitted until a macro is loaded."}, {-307751, "NI VeriStand: The specified operation is not permitted while playing a macro."}, {-307750, "NI VeriStand: Deserialization error. Failed to load macro file."}, {-307749, "NI VeriStand: A simulated DAQ device cannot be used as a Timed Loop timing source or as a chassis master hardware synchronization device."}, {-307748, "NI VeriStand: The VeriStand Engine rebooted while running the system definition file. You must reconnect to the execution host and possibly redeploy the system definition file."}, {-307747, "NI VeriStand: The system definition file contains two targets that are using the same IP address. Each target must have a unique IP address. Only one target can be a Windows target."}, {-307746, "NI VeriStand: The maximum Windows target rate is 1 kHz. To achieve higher rates, use an NI-DAQ device or NI FPGA target."}, {-307745, "NI VeriStand: You must specify a VISA device address for the reflective memory card."}, {-307744, "NI VeriStand: An alarm failed to compile correctly and cannot be executed."}, {-307743, "NI VeriStand: The VeriStand Engine failed to start. A configured start trigger or external timing source did not occur within the specified timeout."}, {-307742, "NI VeriStand: The VeriStand Engine could not be loaded. Make sure that NI VeriStand and the required drivers (such as NI-DAQmx) are installed correctly. Refer to the NI VeriStand readme.html for a list of required software and drivers."}, {-307741, "NI VeriStand: NI VeriStand export data exceeds the allocated reflective memory address."}, {-307740, "NI VeriStand: Invalid data range. The reflective memory network requires a valid address range."}, {-307739, "NI VeriStand: Data on reflective memory must have the correct byte alignment from memory address 0x0."}, {-307738, "NI VeriStand: Unable to share data between two targets. There is not enough dynamic data sharing space."}, {-307737, "NI VeriStand: Unable to create dynamic data sharing between targets. Either the source or destination target does not have a data sharing device."}, {-307736, "NI VeriStand: Unable to share data for the channel. Either the source or destination target does not have reflective memory support."}, {-307735, "NI VeriStand: A required resource is disabled in the current version of the VeriStand Engine. For example, a DAQ board is the master timing device, but the current VeriStand Engine has disabled NI-DAQ. Remove the device or resource from the system definition file."}, {-307734, "NI VeriStand: The scaling and calibration setting is invalid. The channel does not exist or is not scalable."}, {-307733, "NI VeriStand: The version of the calibration file (HardwareCalibrationData.nivscal) is too old to mutate to the current version. Delete the file and manually recreate the calibration settings."}, {-307732, "NI VeriStand: The system has become unresponsive. The Primary Control Loop has been shut down."}, {-307731, "NI VeriStand: The system definition file is not saved in the current version of NI VeriStand."}, {-307730, "NI VeriStand: One or more asynchronous custom devices failed to shut down properly and were aborted by the VeriStand Engine."}, {-307729, "NI VeriStand: The system definition file is missing. Deploy a valid system definition file from the client computer."}, {-307728, "NI VeriStand: One or more channel mappings have incompatible dimensions. Matrix channels only can be mapped to matrix channels with the same dimension."}, {-307727, "NI VeriStand: The requested DAQ device, the master timing source for the timed loop, is unavailable."}, {-307726, "NI VeriStand: A calculated channel failed to compile correctly and cannot be executed."}, {-307725, "NI VeriStand: The value does not match the dimensions of the specified channel."}, {-307724, "NI VeriStand: A DAQ channel initialization VI encountered an unexpected property name."}, {-307723, "NI VeriStand: A property of a DAQ channel has an invalid value. Try changing the value the error message lists. If you used the System Definition API to change the units property of a channel, restore the units to the original value."}, {-307722, "NI VeriStand: A DAQ channel of an unexpected type was found."}, {-307721, "NI VeriStand: Cannot enable Slow Background Conversion Mode if hardware-timed single-point sample mode is disabled for analog input channels. If you want to enable Slow Background Conversion Mode for this device, you must first enable hardware-timed single-point support for its AI channels."}, {-307720, "NI VeriStand: Failed to route PXI_Trig0 from bus segment of chassis master device to other bus segments."}, {-307719, "NI VeriStand: Unable to discover XNET interface(s) before timeout elapsed. Contact National Instruments support at ni.com/support for more information about resolving this error."}, {-307718, "NI VeriStand: Setting Scan Interface mode failed. Before using this mode, make sure NI RIO IO Scan is installed on the target."}, {-307711, "NI VeriStand: A channel and the alias that references it both specify a data source mapping. A channel can only have one data source mapping. Remove the mapping for either the channel or its alias."}, {-307710, "NI VeriStand: The specified item is not an inline custom device. You must pass in a valid reference to an inline custom device."}, {-307704, "NI VeriStand: The specified model is not compatible with the specified execution host."}, {-307703, "NI VeriStand: The specified model is incompatible with NI VeriStand. If you are trying to deploy the model to an RT target, launch the Console Viewer tool to display the console output of the target, which includes information about the source of the error."}, {-307702, "NI VeriStand: The size of the imported model data in the system definition file conflicts with the size in the specified model file. This error can occur if the model file contains a different number of inports, outports, signals, or parameters than when it was imported. This error also can occur if two or more models contain a global parameter with the same name but different dimensions. To correct this error, reload the model in the <b>System Explorer</b> window and verify the dimensions of any global parameters that multiple models contain. Alternatively, change the <b>Scope for Global Parameters</b> option on the <b>Parameters</b> page for a model to <b>Model</b> to avoid conflicts caused when the model shares the global parameter with other models."}, {-307701, "NI VeriStand: Timeout occurred while writing a parameter value to the VeriStand Engine."}, {-307700, "NI VeriStand: One or more Model Execution Loops failed to shut down properly."}, {-307691, "NI VeriStand: Import operation failed for the specified SLSC chassis."}, {-307690, "NI VeriStand: To reconnect to a target without deploying, the restart action for real-time (RT) targets must be set to Run System Definition. To enable the Run System Definition restart action, select the <B>System Initialization</B> node in the <B>System Explorer</B> and select the <B>Run System Definition</B> option button. You must redeploy the system definition to make use of these changes."}, {-307689, "NI VeriStand: The specified target is disabled. Change the target settings in the system definition and redeploy if you wish to use this target."}, {-307688, "NI VeriStand: Timeout occurred while reconnecting a target to the gateway."}, {-307687, "NI VeriStand: The given number of channels and number of values do not match."}, {-307686, "NI VeriStand: The specified target is not defined in the deployed system definition."}, {-307685, "NI VeriStand: Cannot initialize model parameter(s) defined in model parameter file because parameter was not found in system. 1) Ensure the expression of the parameter is spelled correctly in the file. 2) If the file defines a temporary variable, ensure the system definition allows temporary variables. 3) If the file contains aliases, ensure the path to an alias file is correct in the system definition. Verify the contents of the file and the settings  on the <B>Simulation Models</B> configuration page in the <B>System Explorer</B>, and then try again."}, {-307684, "NI VeriStand: Cannot start server because the port address is already in use by another process. To change the port address for the server, select <B>Tools>>Options</B>, browse to the <B>Port Settings</B> page, and change the value of the corresponding control ."}, {-307683, "NI VeriStand: Cannot deploy or connect to the system definition because all targets in the system are disabled. Enable one or more targets in the system definition, and then try to deploy again."}, {-307682, "NI VeriStand: Could not complete one or more requests because a target is offline."}, {-307681, "NI VeriStand: Failed to read the NI VeriStand service configuration file. Repair your NI VeriStand installation to resolve this issue."}, {-307680, "NI VeriStand: An exception occurred when the model parameter file was being parsed."}, {-307679, "NI VeriStand: The VeriStand Gateway is no longer connected to the targets. One of the targets stopped running the system definition file."}, {-307678, "NI VeriStand: The specified workspace tool VI is not open."}, {-307677, "NI VeriStand: The reference to the project file is no longer valid. The referenced project is no longer open."}, {-307676, "NI VeriStand: NI VeriStand cannot open the specified project file because another project is already open."}, {-307675, "NI VeriStand: The VeriStand Gateway cannot complete the specified operation because the number of streamed channels for one or more targets exceeds the maximum size. Stop data logging configurations or graphs to reduce the number of streamed channels. You also can increase the maximum streamed channel count for the targets by editing the system definition file in the <b>System Explorer</b> window."}, {-307674, "NI VeriStand: The Run Workspace function is no longer supported. Use the Connect to System function instead, which has a system definition file parameter instead of a workspace file."}, {-307673, "NI VeriStand: Another VeriStand Gateway already is connected to the execution host. Only one VeriStand Gateway can be connected to an execution host at a time."}, {-307672, "NI VeriStand: One or more targets failed to start within the specified timeout. Verify that any start trigger or clock signals are configured correctly."}, {-307671, "NI VeriStand: The execution host is running a different system definition file than the file specified. You must deploy the system definition file in order to connect to the execution host."}, {-307670, "NI VeriStand: The VeriStand Gateway cannot process the requested operation. The VeriStand Gateway currently is busy performing another operation."}, {-307669, "NI VeriStand: The license is not available, the license is not valid, or NI VeriStand failed to initialize the licensing component."}, {-307668, "NI VeriStand: The specified channel cannot be scaled."}, {-307667, "NI VeriStand: The requested operation on this item reference is invalid."}, {-307666, "NI VeriStand: The specified channel cannot be faulted."}, {-307665, "NI VeriStand: Channel does not have write access."}, {-307664, "NI VeriStand: Channel does not have read access."}, {-307663, "NI VeriStand: Timeout in processing request."}, {-307662, "NI VeriStand: Node is not found in the system."}, {-307661, "NI VeriStand: NI VeriStand failed to deploy the system definition file."}, {-307660, "NI VeriStand: Timeout occurred while deploying a new system definition file."}, {-307659, "NI VeriStand: Invalid password input parameter. The password cannot be an empty string."}, {-307658, "NI VeriStand: NI VeriStand is unable to run the system definition file when a system definition file already is running."}, {-307657, "NI VeriStand: The specified password does not match the current deployed configuration password."}, {-307656, "NI VeriStand: Invalid request. NI VeriStand does not have a system definition file loaded."}, {-307655, "NI VeriStand: Invalid request. NI VeriStand is missing an engine component that is required to process the request."}, {-307654, "NI VeriStand: Cannot perform this request because NI VeriStand is not running a system definition file. Deploy a system definition file, and then try again."}, {-307653, "NI VeriStand: Invalid input file parameter."}, {-307652, "NI VeriStand: Failed to open a connection to NI VeriStand.exe."}, {-307651, "NI VeriStand: The NI VeriStand API does not support this function."}, {-307650, "NI VeriStand: An unexpected error has occurred in the NI VeriStand API."}, {-307617, "NI VeriStand: The system definition contains aliases that are not linked to ny channel. Click on the Error/Warning icon on System Explorer to get a list of aliases that are not linked and either link them to a channel or delete them."}, {-307616, "NI VeriStand: The associated NI-XNET signal has been deleted from the XNET database or it changed so it no longer matches the system definition. If the database no longer contains the signal, delete the signal from the system definition. If the signal changed in the database, reimport the signal."}, {-307615, "NI VeriStand: Cannot set the <B>PXI Backplane Reference Clock</B> for this DAQ device because this device does not support reference-clock synchronization. Select <B>None</B> or <B>Automatic</B>."}, {-307614, "NI VeriStand: The DAQ support files are missing for the channel type selected. Try repairing your installation of NI VeriStand."}, {-307613, "NI VeriStand: You cannot add channels of the type you selected. The DAQ device either contains no channels of this type, or all available channels of this type are already in the system definition."}, {-307612, "NI VeriStand: One or more chassis are unidentified. Open Measurement and Automation Explorer (MAX) and identify the type of the chassis for each controller that is configured in the <b>System 
